vi "TJ's Climber Main.vi"(11 "Control Mode":enum16{"Open", "Forward", "Backward", "Stop"}(ring)) -> ()   [LabVIEW 2018]
uses:
  <vilib>/Rock Robotics/SystemInterfaces/DIO/FPGA_DIOPWMChannel.ctl
  <vilib>/Rock Robotics/WPI/MotorControl/WPI_MotorControlOpen SPARK.vi
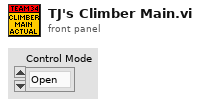
[diagram p1: front panel]
types:
  T1 = typedef "FPGA_DIOPWMChannel.ctl" = enum8{"PWM 0", "PWM 1", "PWM 2", "PWM 3", "PWM 4", "PWM 5", "PWM 6", "PWM 7", "PWM 8", "PWM 9", "PWM MXP 0", "PWM MXP 1", "PWM MXP 2", "PWM MXP 3", "PWM MXP 4", "PWM MXP 5", "PWM MXP 6", "PWM MXP 7", "PWM MXP 8", "PWM MXP 9", "Invalid"}
  T2 = typedef "WPI_MotorControlDeviceRef.ctl" = cluster{"DeviceStatus":errorcluster, "Type":T3, "PWM":cluster{"PWM Channel":T1, "DeadBand":T4}, "CAN":cluster{"Device Number":u8, "SetOutput VI Ref":variant, "GetOutput VI Ref":variant, "Enable VI Ref":variant, "Disable VI Ref":variant, "Data":variant}, "Invert":bool, "DIO PWM":cluster{"PWM \"Enable\" Channel":T1, "DIOChannel":T5, "PWM Rate":dbl}}
  T3 = typedef "WPI_MotorControlType.ctl" = enum16{"PWM", "CAN", "DIO PWM"}
  T4 = typedef "WPI_PWMDeadband.ctl" = cluster{"Name":string, "maxPositivePwm":i32, "minPositivePwm":i32, "centerPwm":i32, "maxNegativePwm":i32, "minNegativePwm":i32, "angularRange":u16}
  T5 = typedef "FPGA_DIOChannel.ctl" = enum8{"DIO 0", "DIO 1", "DIO 2", "DIO 3", "DIO 4", "DIO 5", "DIO 6", "DIO 7", "DIO 8", "DIO 9", "DIO MXP 0", "DIO MXP 1", "DIO MXP 2", "DIO MXP 3", "DIO MXP 4", "DIO MXP 5", "DIO MXP 6", "DIO MXP 7", "DIO MXP 8", "DIO MXP 9", "DIO MXP 10", "DIO MXP 11", "DIO MXP 12", "DIO MXP 13", "DIO MXP 14", "DIO MXP 15", "SPI Port CS1", "SPI Port CS2", "SPI Port CS3", "SPI Port MISO", "SPI Port MOSI", "Invalid"}
  T6 = cluster{"MotorControlDeviceRef":T2, "MotorControlDeviceRef":T2}
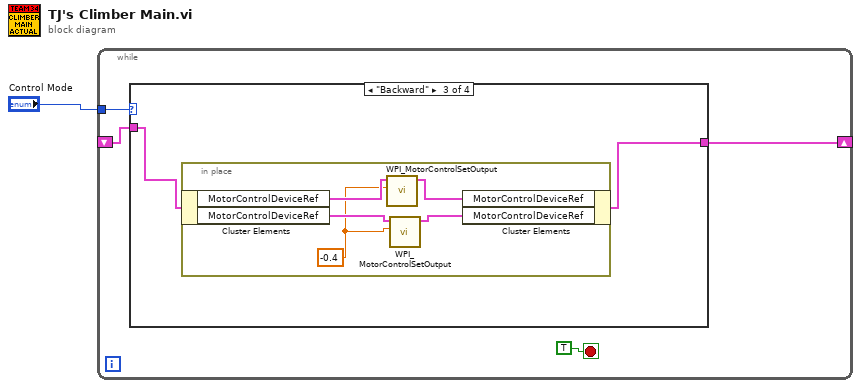
[diagram p0: block diagram]
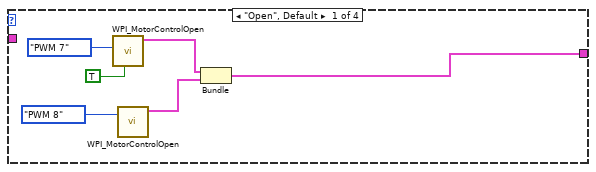
[diagram p2: hidden frame]
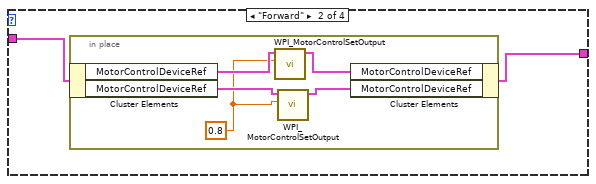
[diagram p3: hidden frame]
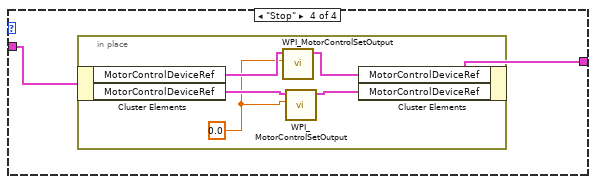
[diagram p4: hidden frame]
diagram:
  n1 = while {
    tunnel: "Control Mode" -> [w5]
    shift-right: [w3] -> _
    shift-left: _ -> [w2]
    stop <- TRUE stop-if-true
    n2 = case shown="\"Backward\"" w5 {
      tunnel: [w8 w12 w19 w26] -> w3
      tunnel: w2 -> [_ w13 w20 w27]
      frame "Open", Default {
        n3 = call-poly <vilib>:"WPI_MotorControlOpen.vi"("Invert"=TRUE, "PWM Channel"=FPGA_DIOPWMChannel."PWM 7") -> ("MotorControlDeviceRef"=w10:T2)  [unwired: 8 in, 1 out]
        n4 = call-poly <vilib>:"WPI_MotorControlOpen.vi"("PWM Channel"=FPGA_DIOPWMChannel."PWM 8") -> ("MotorControlDeviceRef"=w9:T2)  [unwired: 9 in, 1 out]
        n5 = Bundle("MotorControlDeviceRef"=w10, "MotorControlDeviceRef"=w9) -> (w8:T6)  [unwired: 1 in]
      }
      frame "Forward" {
        n6 = in-place {
          w14 = 0.8
          n7 = in-place-cluster #1(w13) -> ("MotorControlDeviceRef"=w18:T2, "MotorControlDeviceRef"=w16:T2)
          n8 = call <vilib>:"WPI_MotorControlSetOutput.vi"("Output"=w14, "MotorControlDevRef"=w18) -> ("MotorControlDevRef"=w17:T2)  [unwired: 7 in, 2 out]
          n9 = call <vilib>:"WPI_MotorControlSetOutput.vi"("Output"=w14, "MotorControlDevRef"=w16) -> ("MotorControlDevRef"=w15:T2)  [unwired: 7 in, 2 out]
          n10 = in-place-cluster #1("MotorControlDeviceRef"=w17, "MotorControlDeviceRef"=w15) -> (w12:T6)
        }
      }
      frame "Backward" {
        n11 = in-place {
          w21 = -0.4
          n12 = in-place-cluster #2(w20) -> ("MotorControlDeviceRef"=w25:T2, "MotorControlDeviceRef"=w23:T2)
          n13 = call <vilib>:"WPI_MotorControlSetOutput.vi"("Output"=w21, "MotorControlDevRef"=w25) -> ("MotorControlDevRef"=w24:T2)  [unwired: 7 in, 2 out]
          n14 = call <vilib>:"WPI_MotorControlSetOutput.vi"("Output"=w21, "MotorControlDevRef"=w23) -> ("MotorControlDevRef"=w22:T2)  [unwired: 7 in, 2 out]
          n15 = in-place-cluster #2("MotorControlDeviceRef"=w24, "MotorControlDeviceRef"=w22) -> (w19:T6)
        }
      }
      frame "Stop" {
        n16 = in-place {
          w28 = 0.0
          n17 = in-place-cluster #3(w27) -> ("MotorControlDeviceRef"=w32:T2, "MotorControlDeviceRef"=w30:T2)
          n18 = call <vilib>:"WPI_MotorControlSetOutput.vi"("Output"=w28, "MotorControlDevRef"=w32) -> ("MotorControlDevRef"=w31:T2)  [unwired: 7 in, 2 out]
          n19 = call <vilib>:"WPI_MotorControlSetOutput.vi"("Output"=w28, "MotorControlDevRef"=w30) -> ("MotorControlDevRef"=w29:T2)  [unwired: 7 in, 2 out]
          n20 = in-place-cluster #3("MotorControlDeviceRef"=w31, "MotorControlDeviceRef"=w29) -> (w26:T6)
        }
      }
    }
  }
